vi "GetSelectedElements.vi"(10 "Masks":bool[](array[boolean]), 11 "Array[in]":dbl[](array[numeric])) -> (3 "Array[out]":dbl[](array[numeric]))   [LabVIEW 2012]
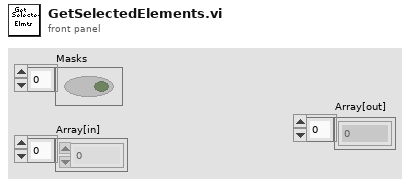
[diagram p1: front panel]
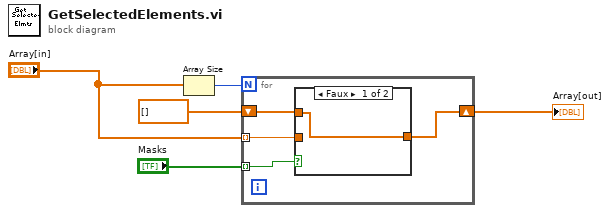
[diagram p0: block diagram]
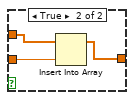
[diagram p2: hidden frame]
diagram:
  n1 = Array Size(array="Array[in]") -> (size(s)=w2:i32)
  n2 = for {
    N: w2 -> [_]
    tunnel: "Array[in]" -> [w8] mode=indexing
    tunnel: "Masks" -> [w9] mode=indexing
    shift-right: [w7] -> w1
    shift-left: dbl[] [] -> [w6]
    n3 = case shown="Faux" w9 {
      tunnel: [w10 w11] -> w7
      tunnel: w8 -> [_ w12]
      tunnel: w6 -> [w10 w13]
      frame False {
      }
      frame True {
        n4 = Insert Into Array(array=w13, new element=w12) -> (w11:dbl[])  [unwired: 1 in]
      }
    }
  }
  "Array[out]" <- w1
